vi "IntakeWheels.vi"(8 "error in":errorcluster, 10 "SensorInputData":T6, 11 "HMI to Control":T2={"RightDriveValue"=0.0, "LeftDriveValue"=0.0, "Arm Manual "=0.0, "Stacker Manual "=0.0, "Claw Manual "=0.0, "ClawSlightOpenNumber"=0, "Intake Value "=0.0, "Arm States"=enum."4 Tote", "Claw States"=enum."Claw Manual ", "Intake Man. or Sense"=enum."Sensing", "Stacker in Manual?"=FALSE, "Drop Stack? "=FALSE, "Tusk Up Request"=FALSE, "Tusk Down Request"=FALSE, "Inver. Wheels  In Request"=FALSE, "Inverse. Wheels Out Request "=FALSE, "Get Out of Manual Control"=FALSE, "Exit Score State"=FALSE, "DriveStraight Help?"=FALSE, "Stacker Shut Off No."=0, "Stacker Need Off?"=FALSE, "Collecting?"=FALSE, "Go to Hover"=FALSE, "Stack Clamp Lock "=FALSE, "Stack Clamp Unlock "=FALSE, "Claw Intake Value "=0.0, "Stack Clamp Lock No. "=0, "Steal Can (ruin their day?)"=FALSE, "Retract (have mercy?)"=FALSE, "Can Grab No. "=0, "Wench Value to Control "=0.0}) -> (0 "error out":errorcluster, 1 "Intake Wheel State Out":T1=enum."Intake Wheels Closed", 2 "SensorInputData Out":T6, 3 "HMI to Control  Out":T2={"RightDriveValue"=0.0, "LeftDriveValue"=0.0, "Arm Manual "=0.0, "Stacker Manual "=0.0, "Claw Manual "=0.0, "ClawSlightOpenNumber"=0, "Intake Value "=0.0, "Arm States"=enum."4 Tote", "Claw States"=enum."Claw Manual ", "Intake Man. or Sense"=enum."Sensing", "Stacker in Manual?"=FALSE, "Drop Stack? "=FALSE, "Tusk Up Request"=FALSE, "Tusk Down Request"=FALSE, "Inver. Wheels  In Request"=FALSE, "Inverse. Wheels Out Request "=FALSE, "Get Out of Manual Control"=FALSE, "Exit Score State"=FALSE, "DriveStraight Help?"=FALSE, "Stacker Shut Off No."=0, "Stacker Need Off?"=FALSE, "Collecting?"=FALSE, "Go to Hover"=FALSE, "Stack Clamp Lock "=FALSE, "Stack Clamp Unlock "=FALSE, "Claw Intake Value "=0.0, "Stack Clamp Lock No. "=0, "Steal Can (ruin their day?)"=FALSE, "Retract (have mercy?)"=FALSE, "Can Grab No. "=0, "Wench Value to Control "=0.0})   [LabVIEW 2014]
uses:
  Typedefs/SensorInputData.ctl
  Typedefs/HMI_to_Control.ctl
  Typedefs/Arm States.ctl
  Typedefs/ClawStates.ctl
  Typedefs/IntakeWheelSenseOrManual.ctl
  Typedefs/IntakeWheelStates.ctl
panel:
  out "Intake Wheel State In":T1=enum."Intake Wheels Closed"
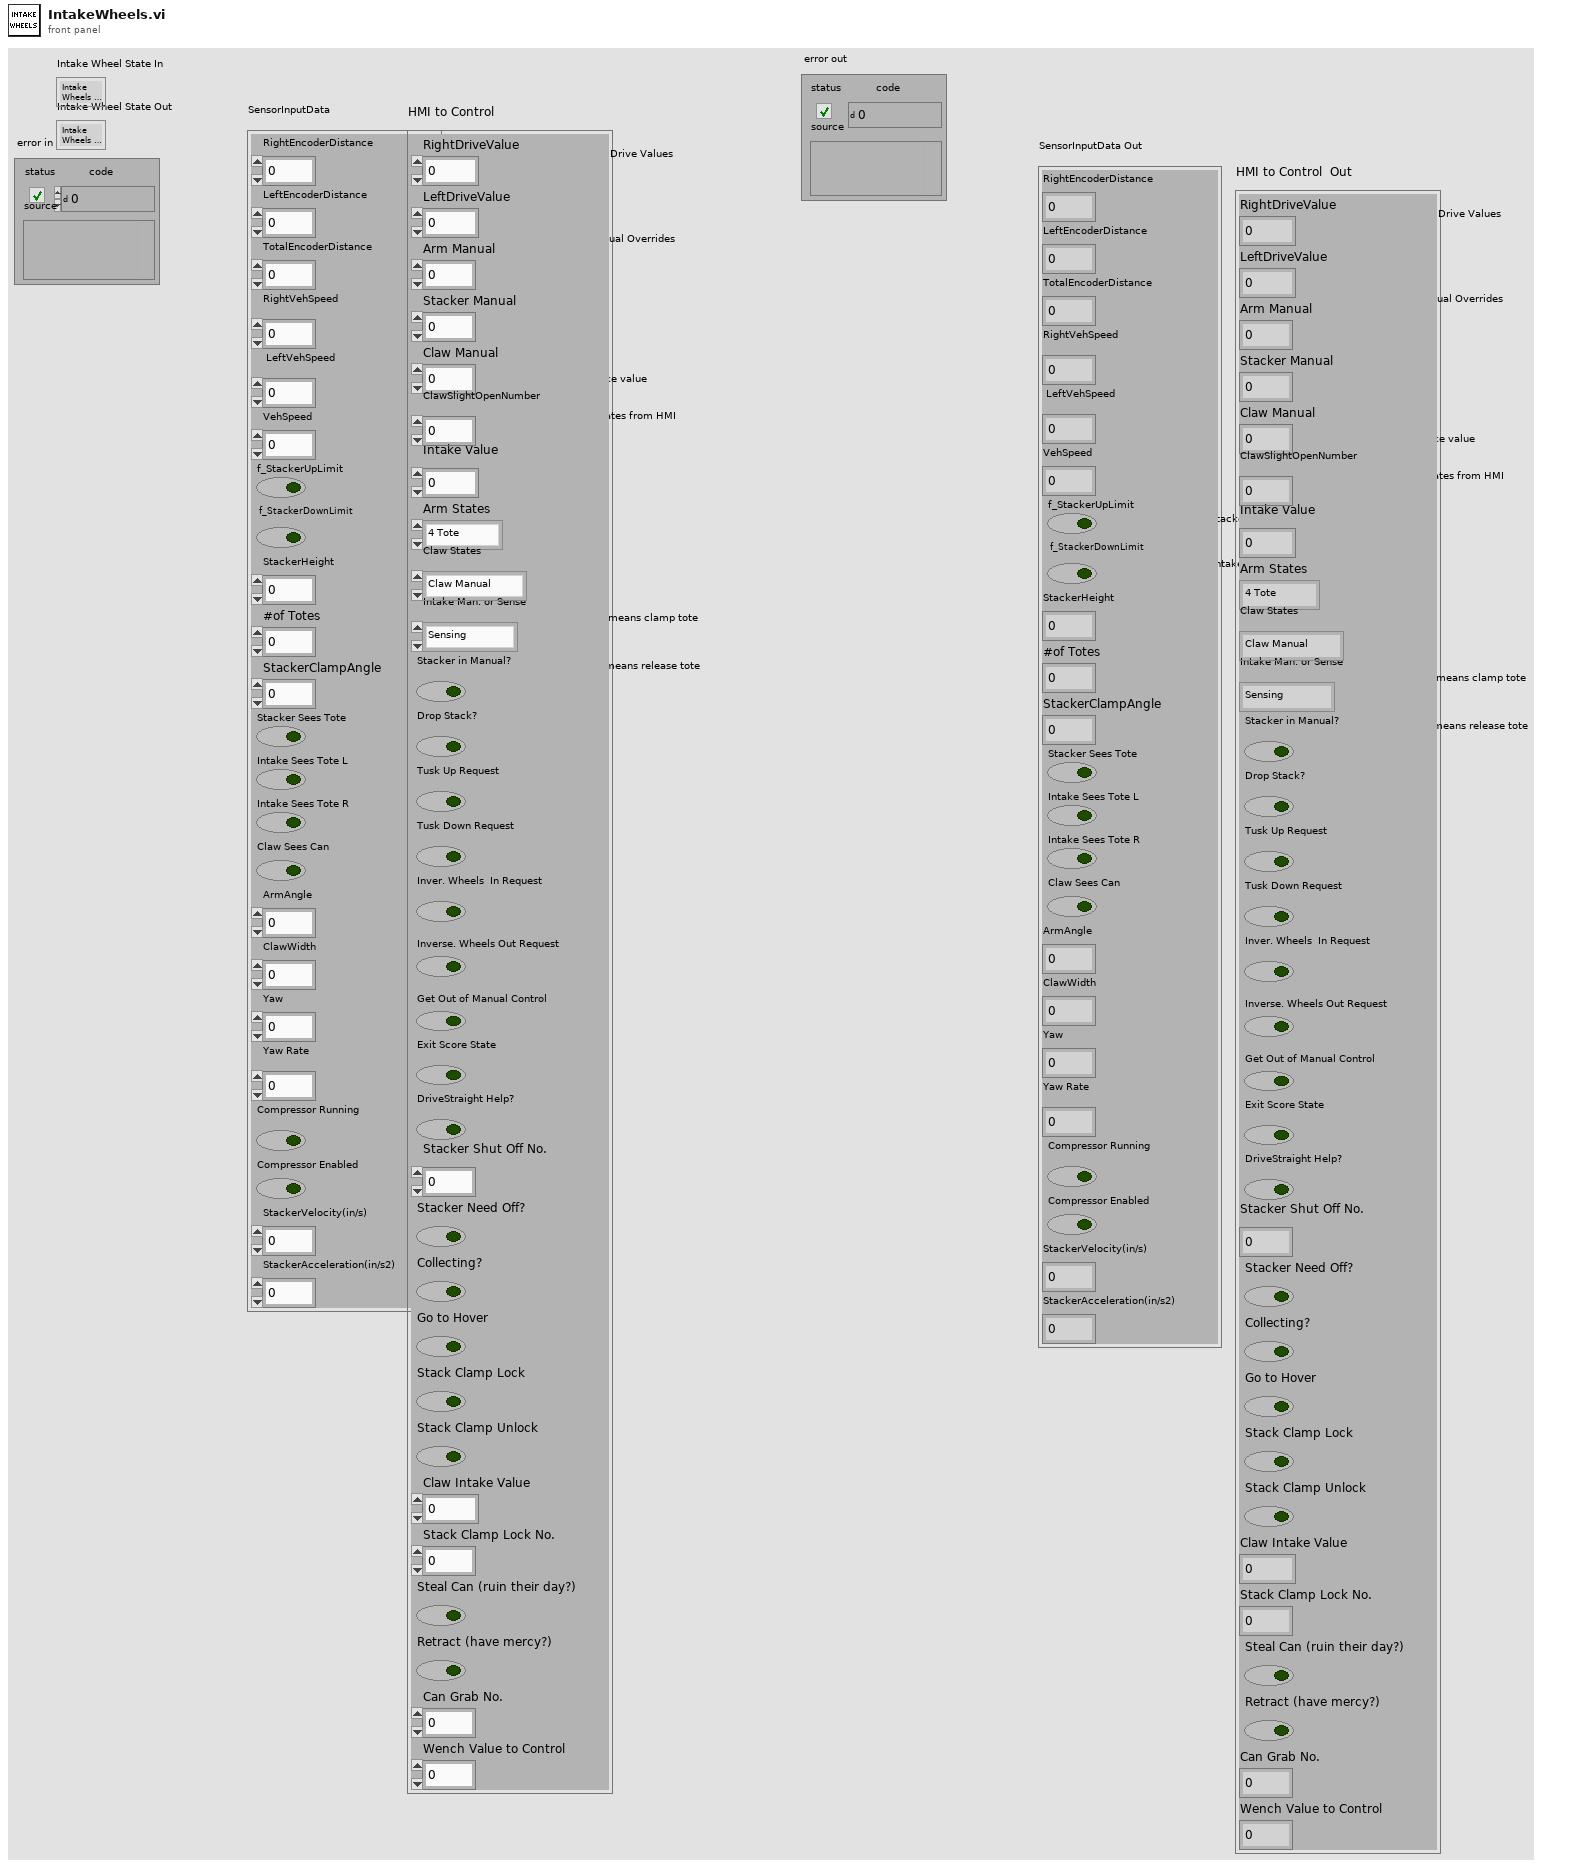
[diagram p1: front panel]
types:
  T1 = typedef "IntakeWheelStates.ctl" = enum16{"Intake Wheels Open", "Intake Wheels Closed", "Decide off of Input", "Delay before Close", "Operator Request"}
  T2 = typedef "HMI_to_Control.ctl" = cluster{"RightDriveValue":dbl, "LeftDriveValue":dbl, "Arm Manual ":dbl, "Stacker Manual ":dbl, "Claw Manual ":dbl, "ClawSlightOpenNumber":i8, "Intake Value ":sgl, "Arm States":T3, "Claw States":T4, "Intake Man. or Sense":T5, "Stacker in Manual?":bool, "Drop Stack? ":bool, "Tusk Up Request":bool, "Tusk Down Request":bool, "Inver. Wheels  In Request":bool, "Inverse. Wheels Out Request ":bool, "Get Out of Manual Control":bool, "Exit Score State":bool, "DriveStraight Help?":bool, "Stacker Shut Off No.":i8, "Stacker Need Off?":bool, "Collecting?":bool, "Go to Hover":bool, "Stack Clamp Lock ":bool, "Stack Clamp Unlock ":bool, "Claw Intake Value ":sgl, "Stack Clamp Lock No. ":i8, "Steal Can (ruin their day?)":bool, "Retract (have mercy?)":bool, "Can Grab No. ":i8, "Wench Value to Control ":dbl}
  T3 = typedef "Arm States.ctl" = enum16{"Arm Manual ", "Ground", "Step", "1 Tote", "2 Tote", "3 Tote", "4 Tote", "5 Tote", "6 Tote", "Flip Can Arm", "Grab Can in auto", "Nudge"}
  T4 = typedef "ClawStates.ctl" = enum16{"Claw Manual ", "Claw Open", "Claw Closed", "Claw Slight Open", "Flip Can"}
  T5 = typedef "IntakeWheelSenseOrManual.ctl" = enum16{"Sensing", "Manual "}
  T6 = typedef "SensorInputData.ctl" = cluster{"RightEncoderDistance":dbl, "LeftEncoderDistance":dbl, "TotalEncoderDistance":dbl, "RightVehSpeed":dbl, "LeftVehSpeed":dbl, "VehSpeed":dbl, "f_StackerUpLimit":bool, "f_StackerDownLimit":bool, "StackerHeight":dbl, "#of Totes":u8, "StackerClampAngle":dbl, "Stacker Sees Tote":bool, "Intake Sees Tote L":bool, "Intake Sees Tote R":bool, "Claw Sees Can":bool, "ArmAngle":dbl, "ClawWidth":dbl, "Yaw":dbl, "Yaw Rate":dbl, "Compressor Running":bool, "Compressor Enabled":bool, "StackerVelocity(in/s)":dbl, "StackerAcceleration(in/s2)":dbl}
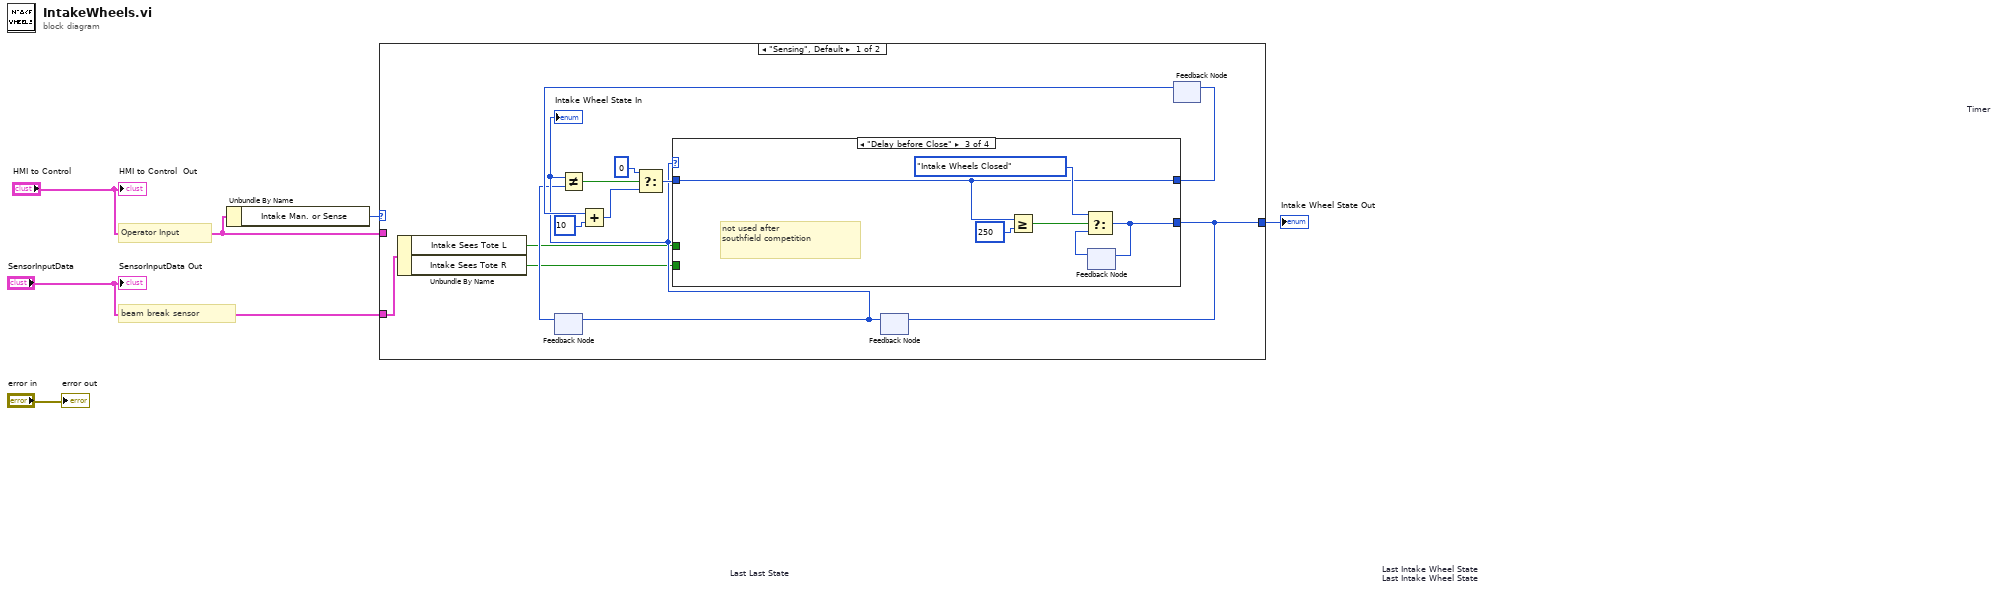
[diagram p0: block diagram]
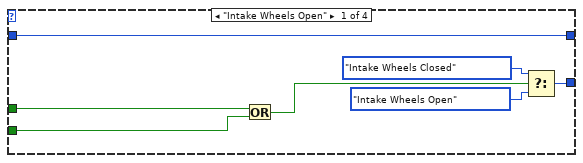
[diagram p2: hidden frame]
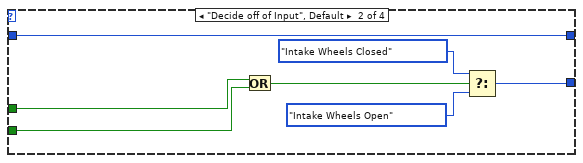
[diagram p3: hidden frame]
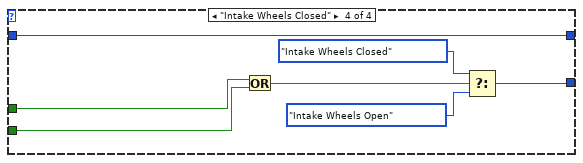
[diagram p4: hidden frame]
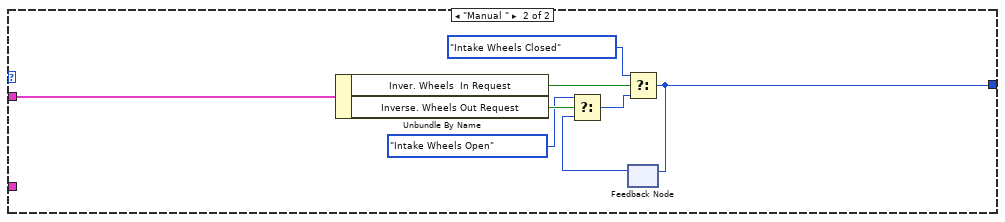
[diagram p5: hidden frame]
diagram:
  # "Operator Input"
  # "beam break sensor"
  n1 = Unbundle By Name("HMI to Control") -> ("Intake Man. or Sense"=w2:T5)
  n2 = case shown="\"Sensing\", Default" w2 {
    tunnel: "SensorInputData" -> [w18 _]
    tunnel: "HMI to Control" -> [_ w53]
    tunnel: [w7 w47] -> w1
    frame "Sensing", Default {
      n3 = Unbundle By Name(w18) -> ("Intake Sees Tote L"=w8:bool, "Intake Sees Tote R"=w6:bool)
      n4 = feedback #1 "Last Last State"() -> (w9:T1)  [unwired: 1 in]
      n5 = feedback #2 "Last Intake Wheel State\nLast Intake Wheel State"() -> (w10:T1)  [unwired: 1 in]
      "Intake Wheel State In" <- w10
      n6 = feedback-in #1(w10) -> ()
      n7 = Not Equal?(x=w10, y=w9) -> (x != y?=w17:bool)
      n8 = feedback #3 "Timer"() -> (w13:u32)  [unwired: 1 in]
      n9 = Add(x=w13, y=u32 10) -> (x+y=w11:u32)
      n10 = Select(t=u32 0, s=w17, f=w11) -> (s? t:f=w14:u32)
      n11 = case shown="\"Delay before Close\"" w10 {
        tunnel: w8 -> [w21 w28 _ w41]
        tunnel: [w23 w29 w35 w43] -> w7
        tunnel: [w25 w32 w36 w44] -> w15
        tunnel: w14 -> [w25 w32 w36 w44]
        tunnel: w6 -> [w19 w27 _ w39]
        frame "Intake Wheels Open" {
          n12 = Or(x=w21, y=w19) -> (x .or. y?=w20:bool)
          n13 = Select(t=IntakeWheelStates."Intake Wheels Closed" ("Intake Wheel States"), s=w20, f=IntakeWheelStates."Intake Wheels Open") -> (s? t:f=w23:T1)
        }
        frame "Decide off of Input", Default {
          n14 = Or(x=w28, y=w27) -> (x .or. y?=w26:bool)
          n15 = Select(t=IntakeWheelStates."Intake Wheels Closed" ("Intake Wheel States"), s=w26, f=IntakeWheelStates."Intake Wheels Open" ("Intake Wheel States")) -> (s? t:f=w29:T1)
        }
        frame "Delay before Close" {
          # "not used after\nsouthfield competition"
          n16 = Greater Or Equal?(x=w36, y=u32 250) -> (x >= y?=w33:bool)
          n17 = feedback #4() -> (w34:T1)  [unwired: 1 in]
          n18 = Select(t=IntakeWheelStates."Intake Wheels Closed" ("Intake Wheel States"), s=w33, f=w34) -> (s? t:f=w35:T1)
          n19 = feedback-in #4(w35) -> ()
        }
        frame "Intake Wheels Closed" {
          n20 = Or(x=w41, y=w39) -> (x .or. y?=w40:bool)
          n21 = Select(t=IntakeWheelStates."Intake Wheels Closed" ("Intake Wheel State In 2"), s=w40, f=IntakeWheelStates."Intake Wheels Open") -> (s? t:f=w43:T1)
        }
      }
      n22 = feedback-in #2(w7) -> ()
      n23 = feedback-in #3(w15) -> ()
    }
    frame "Manual " {
      n24 = Unbundle By Name(w53) -> ("Inver. Wheels  In Request"=w51:bool, "Inverse. Wheels Out Request"=w52:bool)
      n25 = feedback #5() -> (w46:T1)  [unwired: 1 in]
      n26 = Select(t=IntakeWheelStates."Intake Wheels Open" ("Intake Wheel States"), s=w52, f=w46) -> (s? t:f=w48:T1)
      n27 = Select(t=IntakeWheelStates."Intake Wheels Closed" ("Intake Wheel States"), s=w51, f=w48) -> (s? t:f=w47:T1)
      n28 = feedback-in #5(w47) -> ()
    }
  }
  "Intake Wheel State Out" <- w1
  "SensorInputData Out" <- "SensorInputData"
  "HMI to Control  Out" <- "HMI to Control"
  "error out" <- "error in"
